vi "main interface.vi"() -> ()   [LabVIEW 2022 SP3]
uses:
  <vilib>/Utility/file.llb/Write Delimited Spreadsheet (string).vi
  <vilib>/httpClient/LabVIEWHTTPClient.lvlib
panel:
  in  "Tab Control":enum32{"Page 1", "Page 2"}(tab)
  in  "Lock Button":bool
  in  "Password":string
  in  "Username":string
  in  "file path (dialog if empty)":path
  out "Niveau de chlore":string
  out "Niveau de conductivité":string
  out "Conductivité":dbl(knob) scale=0.0..500.0
  out "Etat de l'eau":string
  out "Alerte":bool
  out "message d'alerte":string
  out "Turbidité":dbl(knob) scale=0.0..100.0
  out "Niveau de turbidité":string
  out "Niveau de PH":string
  out "PH Level":dbl(knob) scale=0.0..14.0
  out "Chlore":dbl(knob) scale=0.0..5.0
  out "Niveau de TDS":string
  out "TDS":dbl(knob) scale=0.0..500.0
  in  "stop":bool
  # "système de contrôle de qualité d'eau"
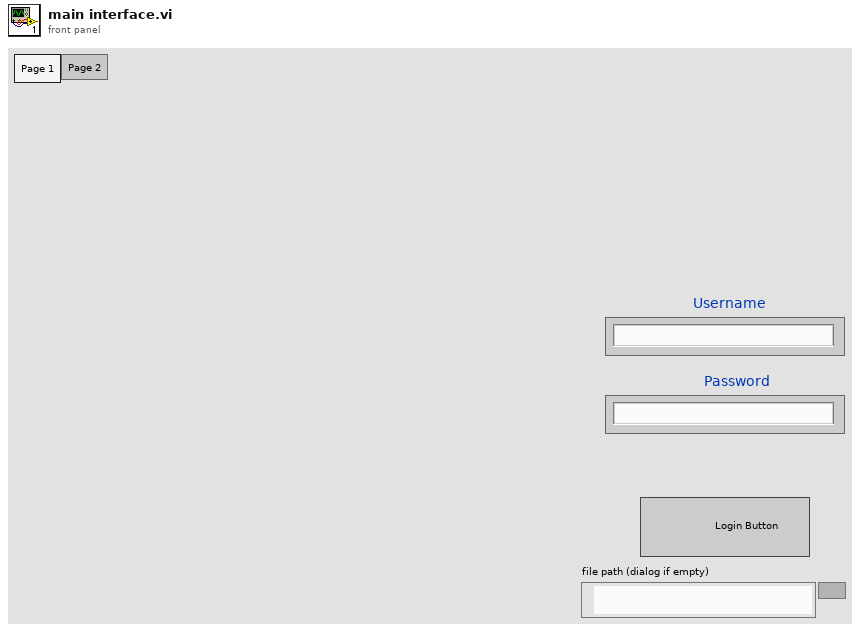
[diagram p1: front panel]
types:
  T1 = typedef "LabVIEWHTTPClient.lvlib/ClientHandle.ctl" = refnum<k1>
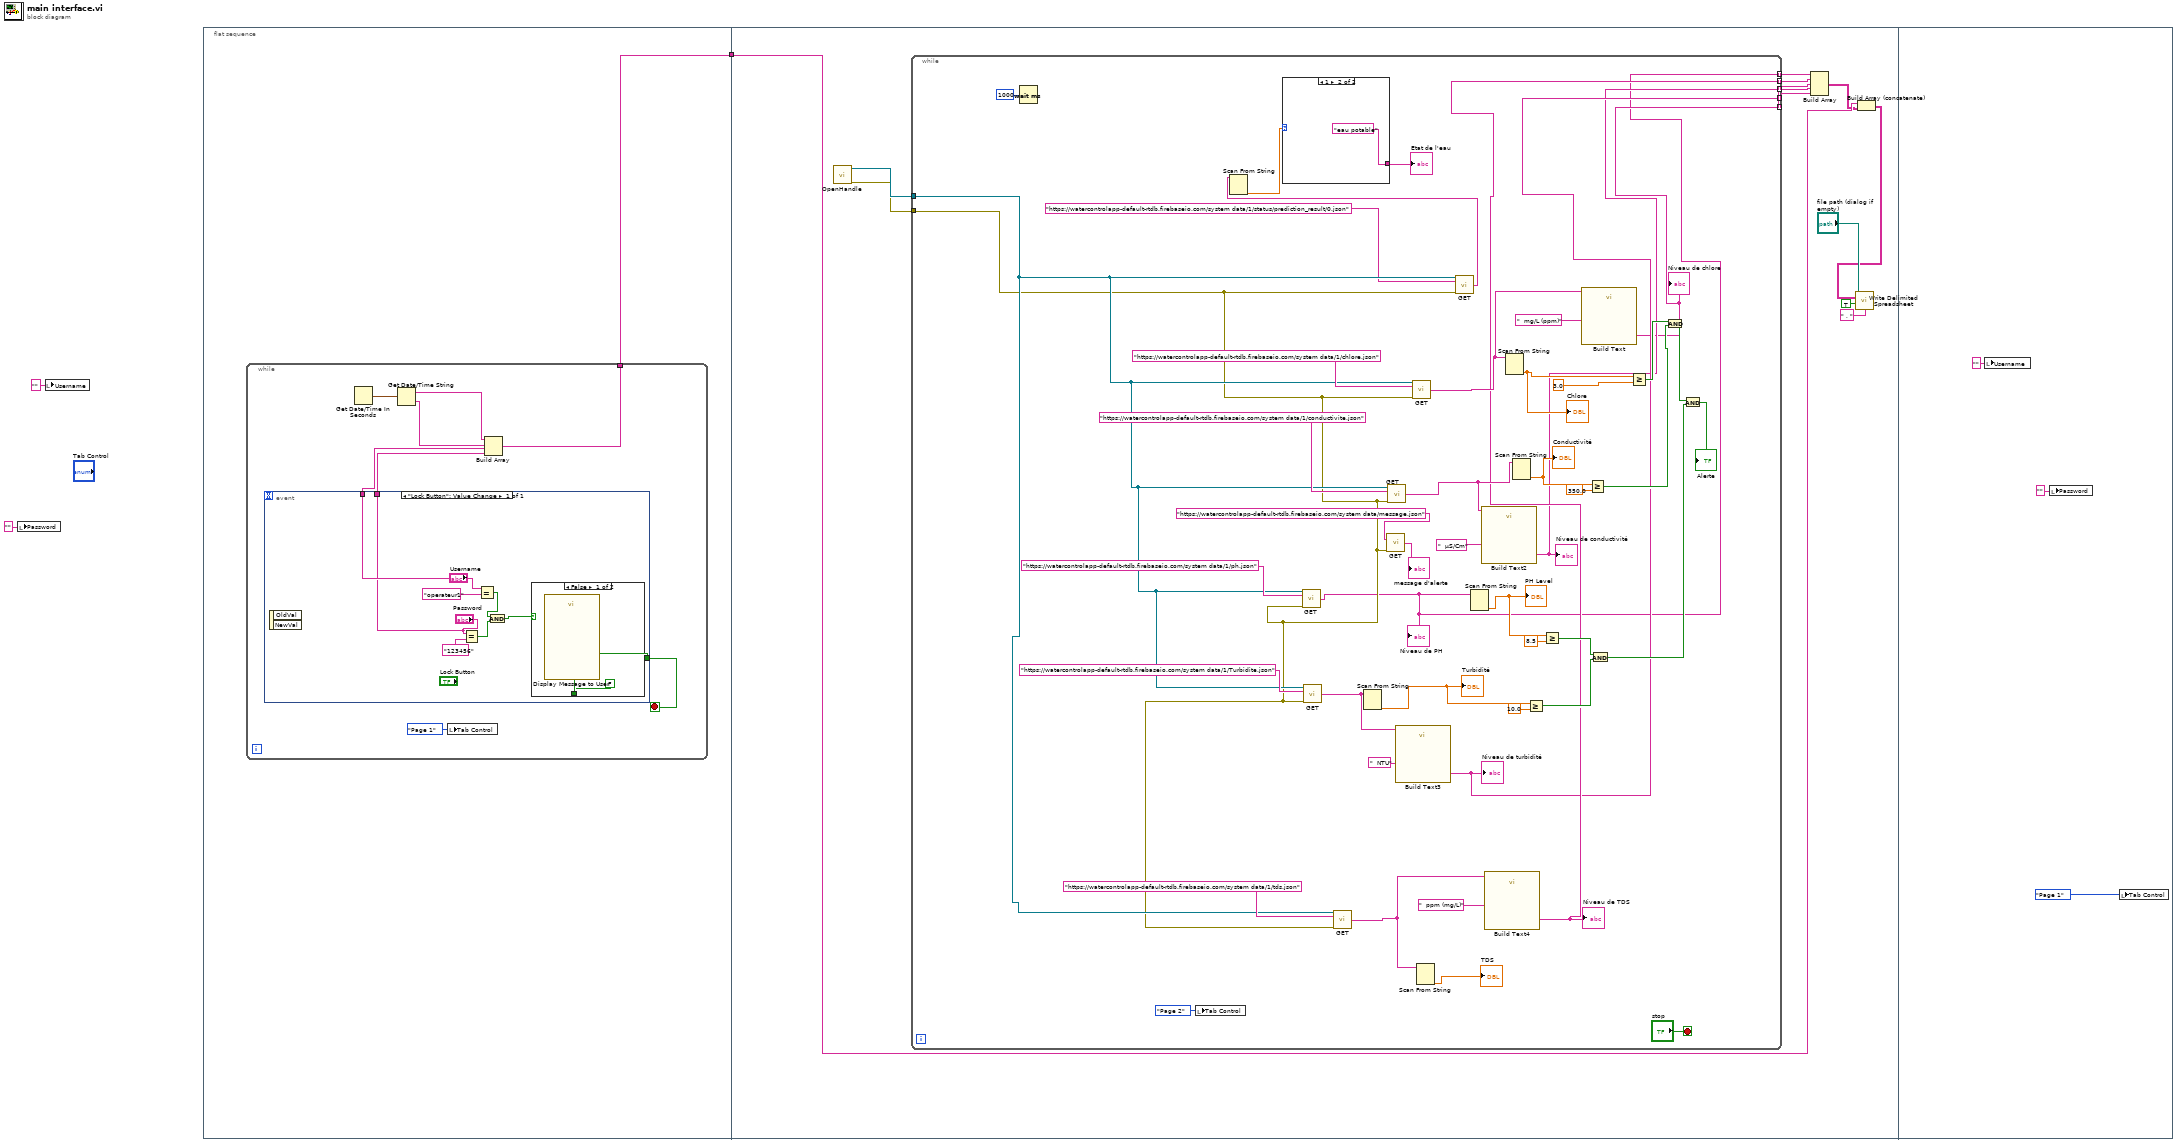
[diagram p0: block diagram]
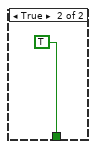
[diagram p2: hidden frame]
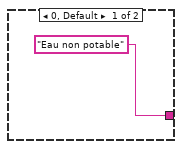
[diagram p3: hidden frame]
diagram:
  n1 = local write "Password"("" ("Password")) -> ()
  n2 = local write "Username"("" ("Username")) -> ()
  n3 = flat-sequence {
    tunnel: [w4] -> w1
    tunnel: w1 -> [w27]
    frame #0 {
      n4 = while {
        tunnel: [w5] -> w4
        stop <- w12 stop-if-true
        n5 = event shown="[0] \"Lock Button\": Value Change" {
          selector: _ -> [_]
          dyn-events: _ -> [_]
          timeout: _ -> [_]
          tunnel: [w15] -> w12
          tunnel: ["Username"] -> w9
          tunnel: ["Password"] -> w10
          event "Lock Button": Value Change {
            n6 = event-data() -> ()  [unwired: 1 in, 2 out]
            n7 = Equal?(x="Password", y="123456") -> (x = y?=w17:bool)
            n8 = Equal?(x="Username", y="operateur1") -> (x = y?=w18:bool)
            n9 = And(x=w18, y=w17) -> (x .and. y?=w16:bool)
            n10 = case shown="False" w16 {
              tunnel: [FALSE TRUE] -> w15
              frame False {
                n11 = call "Display Message to User"() -> ()  [unwired: 10 in, 2 out]
              }
              frame True {
              }
            }
          }
        }
        n12 = Get Date/Time In Seconds() -> (seconds since 1Jan1904=w8:timestamp)
        n13 = Get Date/Time String(seconds (now)=w8) -> (date string=w6:string, time string=w7:string)  [unwired: 2 in]
        n14 = local write "Tab Control"(enum32{"Page 1", "Page 2"}."Page 1" ("Tab Control")) -> ()
        n15 = Build Array(w6, w7, w9, w10) -> (w5:string[])
      }
    }
    frame #1 {
      n16 = call <vilib>:"OpenHandle.vi"() -> ("client handle out"=w35:T1, "error out"=w34:errorcluster)  [unwired: 14 in]
      n17 = while {
        tunnel: w35 -> [w48]
        tunnel: w34 -> [w47]
        tunnel: [w41] -> w33 mode=indexing
        tunnel: [w45] -> w32 mode=indexing
        tunnel: [w42] -> w31 mode=indexing
        tunnel: [w43] -> w30 mode=indexing
        tunnel: [w44] -> w29 mode=indexing
        stop <- "stop" stop-if-true
        n18 = Wait (ms)(milliseconds to wait=u32 1000) -> ()  [unwired: 1 out]
        n19 = local write "Tab Control"(enum32{"Page 1", "Page 2"}."Page 2" ("Tab Control")) -> ()
        n20 = call <vilib>:"GET.vi"("client handle"=w48, "url"="https://watercontrolapp-default-rtdb.firebaseio.com/system data/1/ph.json", "error in (no error)"=w47) -> ("body"=w41:string)  [unwired: 9 in, 3 out]
        "Niveau de PH" <- w41
        n21 = call <vilib>:"GET.vi"("client handle"=w48, "url"="https://watercontrolapp-default-rtdb.firebaseio.com/system data/1/Turbidite.json", "error in (no error)"=w47) -> ("body"=w50:string)  [unwired: 9 in, 3 out]
        n22 = call <vilib>:"GET.vi"("client handle"=w48, "url"="https://watercontrolapp-default-rtdb.firebaseio.com/system data/1/tds.json" ("url 2"), "error in (no error)"=w47) -> ("body"=w54:string)  [unwired: 9 in, 3 out]
        n23 = Scan From String(input string=w50) -> (output 1=w65:dbl)  [unwired: 4 in, 3 out]
        "Turbidité" <- w65
        n24 = call <vilib>:"GET.vi"("url"="https://watercontrolapp-default-rtdb.firebaseio.com/system data/message.json", "error in (no error)"=w47) -> ("body"=→"message d'alerte":string)  [unwired: 10 in, 3 out]
        n25 = call <vilib>:"GET.vi"("client handle"=w48, "url"="https://watercontrolapp-default-rtdb.firebaseio.com/system data/1/conductivite.json" ("url 3"), "error in (no error)"=w47) -> ("body"=w52:string)  [unwired: 9 in, 3 out]
        n26 = call "Build Text3"("Beginning Text"=w50, "turbidité"="  NTU") -> ("Result"=w44:string)  [unwired: 12 in, 1 out]
        "Niveau de turbidité" <- w44
        n27 = call <vilib>:"GET.vi"("client handle"=w48, "url"="https://watercontrolapp-default-rtdb.firebaseio.com/system data/1/chlore.json" ("url 2"), "error in (no error)"=w47) -> ("body"=w51:string)  [unwired: 9 in, 3 out]
        n28 = Scan From String(input string=w54) -> (output 1=→"TDS":dbl)  [unwired: 4 in, 3 out]
        n29 = call <vilib>:"GET.vi"("client handle"=w48, "url"="https://watercontrolapp-default-rtdb.firebaseio.com/system data/1/status/prediction_result/0.json", "error in (no error)"=w47) -> ("body"=w38:string)  [unwired: 9 in, 3 out]
        n30 = Scan From String(input string=w38) -> (output 1=w37:dbl)  [unwired: 4 in, 3 out]
        n31 = case shown="1" w37 {
          tunnel: ["Eau non potable" "eau potable"] -> w36
          frame 0, Default {
          }
          frame 1 {
          }
        }
        "Etat de l'eau" <- w36
        n32 = Scan From String(input string=w41) -> (output 1=w63:dbl)  [unwired: 4 in, 3 out]
        "PH Level" <- w63
        n33 = call "Build Text2"("Beginning Text"=w52, "conductivité"="  µS/Cm") -> ("Result"=w43:string)  [unwired: 12 in, 1 out]
        "Niveau de conductivité" <- w43
        n34 = call "Build Text4"("Beginning Text"=w54, "tds"="  ppm (mg/L)") -> ("Result"=w45:string)  [unwired: 12 in, 1 out]
        "Niveau de TDS" <- w45
        n35 = Scan From String(input string=w51) -> (output 1=w57:dbl)  [unwired: 4 in, 3 out]
        "Chlore" <- w57
        n36 = Scan From String(input string=w52) -> (output 1=w69:dbl)  [unwired: 4 in, 3 out]
        "Conductivité" <- w69
        n37 = Greater Or Equal?(x=w65, y=10.0) -> (x >= y?=w60:bool)
        n38 = Greater Or Equal?(x=w63, y=8.5) -> (x >= y?=w61:bool)
        n39 = call "Build Text"("Beginning Text"=w51, "chlore"="  mg/L (ppm)") -> ("Result"=w42:string)  [unwired: 12 in, 1 out]
        "Niveau de chlore" <- w42
        n40 = Greater Or Equal?(x=w69, y=350.0) -> (x >= y?=w74:bool)
        n41 = And(x=w61, y=w60) -> (x .and. y?=w58:bool)
        n42 = Greater Or Equal?(x=w57, y=3.0) -> (x >= y?=w75:bool)
        n43 = And(x=w75, y=w74) -> (x .and. y?=w59:bool)
        n44 = And(x=w59, y=w58) -> (x .and. y?=→"Alerte":bool)
      }
      n45 = Build Array(w33, w32, w31, w30, w29) -> (w26:string[][])
      n46 = Build Array (concatenate)(w27, w26) -> (w25:string[][])
      n47 = call-poly <vilib>:"Write Delimited Spreadsheet.vi"("file path (dialog if empty)"="file path (dialog if empty)", "2D data"=w25, "append to file? (new file:F)"=TRUE, "delimiter (\\t)"=" , " ("delimiter (\\t)")) -> ()  [unwired: 10 in, 2 out]
    }
    frame #2 {
      n48 = local write "Username"("" ("Username")) -> ()
      n49 = local write "Password"("" ("Password")) -> ()
      n50 = local write "Tab Control"(enum32{"Page 1", "Page 2", "Page 3"}."Page 1" ("Tab Control")) -> ()
    }
  }
